vi "Send Command.vi"(8 "error in (no error)":errorcluster, 10 "Command":string="cPPS\r", 11 "Serial Port In":refnum<visa-resource-name>) -> (0 "error out":errorcluster, 2 "Response":string, 3 "Serial Port Out":refnum<visa-resource-name>)   [LabVIEW 2015, in "Eclipse TI.lvlib" / "Eclipse TI.lvclass"]
uses:
  Eclipse TI.lvclass
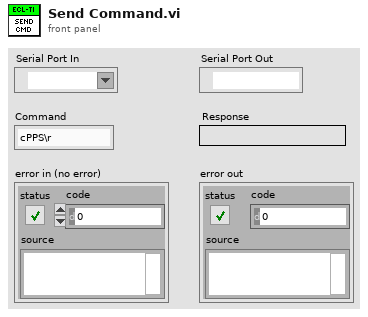
[diagram p1: front panel]
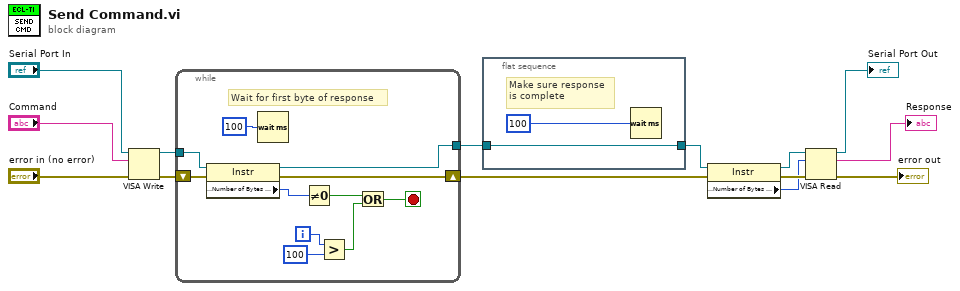
[diagram p0: block diagram]
diagram:
  n1 = VISA Write(VISA resource name="Serial Port In", write buffer="Command", error in (no error)="error in (no error)") -> (VISA resource name out=w6:refnum<visa-resource-name>, error out=w10:errorcluster)  [unwired: 1 out]
  n2 = while {
    tunnel: w6 -> [w25]
    tunnel: [w24] -> w7
    shift-right: [w16] -> w12
    shift-left: w10 -> [w17]
    i -> [w18]
    stop <- w21 stop-if-true
    # "Wait for first byte of response"
    n3 = property class="Instr"(reference=w25, error in=w17) -> (reference out=w24:refnum<visa-resource-name>, error out=w16:errorcluster, "Serial Settings:Number of Bytes at Serial Port"=w23:u32)
    n4 = Wait (ms)(milliseconds to wait=u32 100) -> ()  [unwired: 1 out]
    n5 = Not Equal To 0?(x=w23) -> (x != 0?=w20:bool)
    n6 = Greater?(x=w18, y=100) -> (0:w19:bool)
    n7 = Or(x=w20, y=w19) -> (x .or. y?=w21:bool)
  }
  n8 = flat-sequence {
    tunnel: [w26] -> w1
    tunnel: w7 -> [w26]
    frame #0 {
      # "Make sure response\nis complete"
      n9 = Wait (ms)(milliseconds to wait=u32 100) -> ()  [unwired: 1 out]
    }
  }
  n10 = property class="Instr"(reference=w1, error in=w12) -> (reference out=w3:refnum<visa-resource-name>, error out=w13:errorcluster, "Serial Settings:Number of Bytes at Serial Port"=w2:u32)
  n11 = VISA Read(VISA resource name=w3, byte count=w2, error in (no error)=w13) -> (VISA resource name out=→"Serial Port Out":refnum<visa-resource-name>, read buffer=→"Response":string, error out=→"error out":errorcluster)  [unwired: 1 out]
